vi "data convert.vi"(8 "error in (no error)":errorcluster caption="错误输入（无错误）", 11 "Primary Productivity 输入":refnum<class "Primary Productivity.lvclass">) -> (0 "error out":errorcluster caption="错误输出", 2 "data":T1, 3 "Primary Productivity 输出":refnum<class "Primary Productivity.lvclass">)   [LabVIEW 2016, in "Primary Productivity.lvclass"]
uses:
  Primary Productivity.lvclass
  Primary Productivity.lvclass/Primary Productivity.ctl
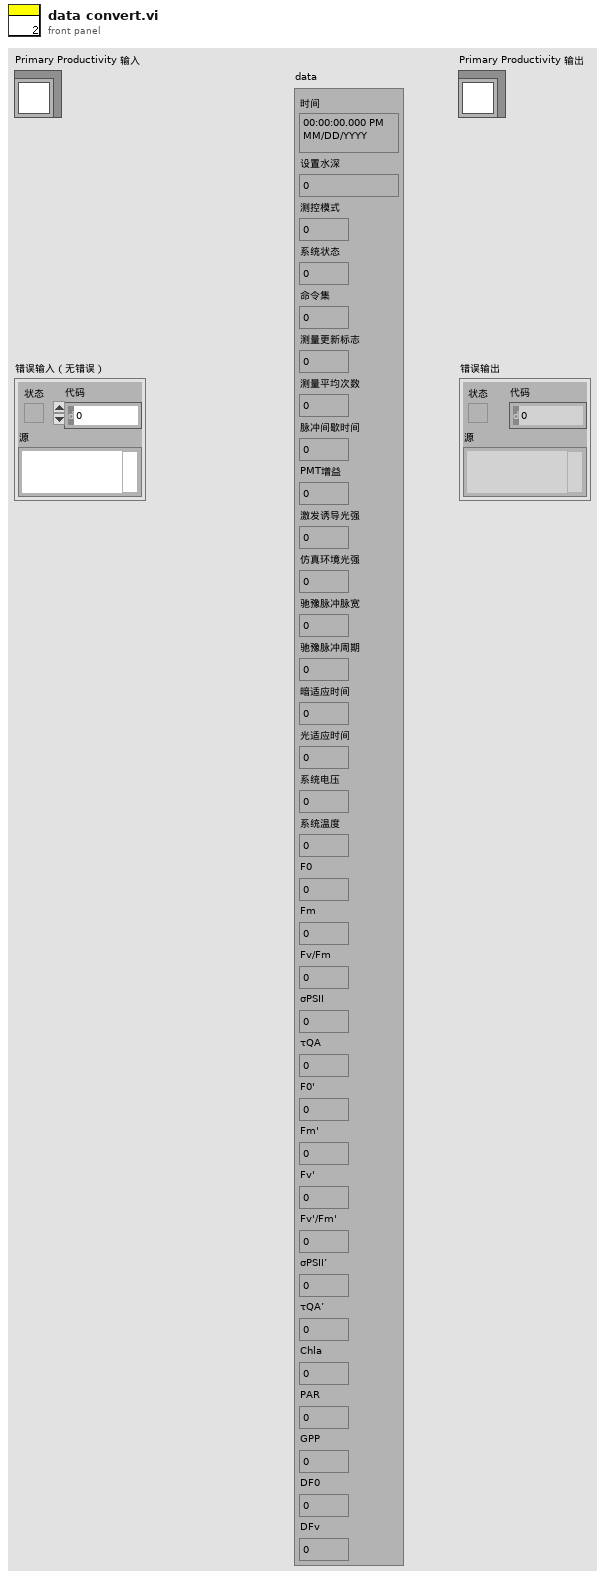
[diagram p1: front panel]
types:
  T1 = cluster{"时间":timestamp, "设置水深":sgl, "测控模式":u16, "系统状态":u16, "命令集":u16, "测量更新标志":u16, "测量平均次数":u16, "脉冲间歇时间":u16, "PMT增益":u16, "激发诱导光强":u16, "仿真环境光强":u16, "驰豫脉冲脉宽":u16, "驰豫脉冲周期":u16, "暗适应时间":u16, "光适应时间":u16, "系统电压":sgl, "系统温度":sgl, "F0":sgl, "Fm":sgl, "Fv/Fm":sgl, "σPSII":sgl, "τQA":sgl, "F0'":sgl, "Fm'":sgl, "Fv'":sgl, "Fv'/Fm'":sgl, "σPSII’":sgl, "τQA’":sgl, "Chla":sgl, "PAR":sgl, "GPP":sgl, "DF0":sgl, "DFv":sgl}
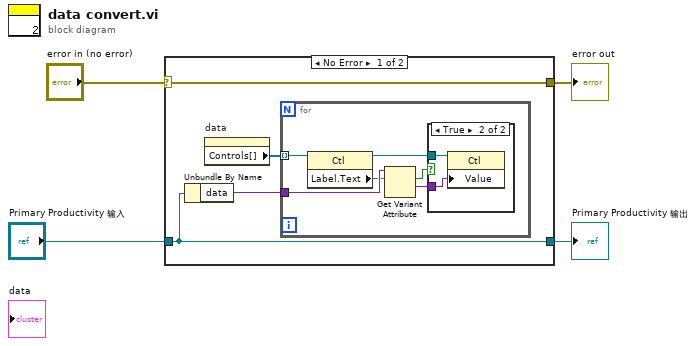
[diagram p0: block diagram]
diagram:
  n1 = case shown="No Error" "error in (no error)" {
    selector: "error in (no error)" -> [w8 w18]
    tunnel: [w8 w18] -> w3
    tunnel: [w7 w17] -> w1
    tunnel: "Primary Productivity 输入" -> [w7 w17]
    frame No Error {
      n2 = Unbundle By Name(w7) -> ("data"=w6:variant)
      n3 = property on="data" class="Clust (strict)"() -> ("Controls[]"=w5:refnum<vi>[])  [unwired: 2 in, 2 out]
      n4 = for {
        tunnel: w6 -> [w14]
        tunnel: w5 -> [w13] mode=indexing
        n5 = property class="Ctl"(reference=w13) -> (reference out=w12:refnum<vi>, "Label.Text"=w10:string)  [unwired: 1 in, 1 out]
        n6 = Get Variant Attribute(Variant=w14, name=w10) -> (found=w11:bool, value=w9:variant)  [unwired: 2 in, 2 out]
        n7 = case shown="True" w11 {
          tunnel: w12 -> [_ w16]
          tunnel: w9 -> [_ w15]
          frame False {
          }
          frame True {
            n8 = property class="Ctl"(reference=w16, "Value"=w15) -> ()  [unwired: 1 in, 2 out]
          }
        }
      }
    }
    frame Error {
    }
  }
  "error out" <- w3
  "Primary Productivity 输出" <- w1
